vi "Acquire Sound.vi"() -> (0 "DAQ Error":errorcluster)   [LabVIEW 2021]
uses:
  Sub_vis/Upload Data.ctl
  Globals/Meas_global.vi
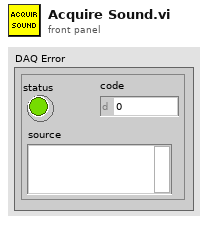
[diagram p1: front panel]
types:
  T1 = typedef "Setup.ctl" = enum16{"Run Program", "Show Setup", "Save Current Setup", "Setup Front Panel"}
  T2 = typedef "Upload Data.ctl" = enum16{"Voltage Array", "Time Trace Cluster"}
  T3 = typedef "Analysis_info_cluster.ctl" = cluster{"Colour":u32, "Inst type":T4, "Inst name":string, "Symbol":string, "Code name":string, "Extra Info":string, "Inst Array":T5, "Extra Titles":string[], "Extra Values":string[], "U":dbl, "u^2":dbl, "u^3":dbl, "u^4":dbl, "Skew_u":dbl, "Kurt_u":dbl, "Sd Error in Mean":dbl, "% u'/U":dbl, "X":dbl, "Y":dbl, "Z":dbl, "Timescale integral Estimate":dbl, "Sd Error in Variance":dbl, "Calib File":path, "Calib Constants":dbl[], "Output Position":bool, "Stats":enum16{"None", "Basic", "Full"}, "Av Sampling Rate":dbl, "Av No of Samples":dbl, "Total Meas Time (s)":dbl, "ADAM Ch Name":string, "Max value":dbl, "Min value":dbl, "Req Sample Rate Hz":dbl, "Sync Delay Time (s)":dbl, "Ch No":i16, "Device":string, "Use Latest Calib":bool, "Port":string, "Metadata Ch Names":string[], "Metadata Ch Values":string[], "Label":string}
  T4 = typedef "Inst_type.ctl" = enum16{"Raw voltage", "Raw with zero offsetting", "Propeller anemometer", "Pressure Transducer", "Pitot-static tube", "Hot wire", "Cross wire 1", "Cross wire 2", "Generic Linear", "Generic Polynomial", "Generic BackPoly", "Fast FID", "Thermocouple", "Cold wire", "Pulsed Wire", "LDA Vel", "LDA Tran time", "LDA Arr time", "Microphone"}
  T5 = typedef "Instrument_Array.ctl" = enum16{"PWA", "LDA", "Analogue"}
  T6 = typedef "Device ID port info.ctl" = cluster{"Ch No":i16[], "Req Sampling Rate":dbl[], "Port":string, "Index":i32[]}
  T7 = typedef "Rendezvous RefNum" = refnum<k1>
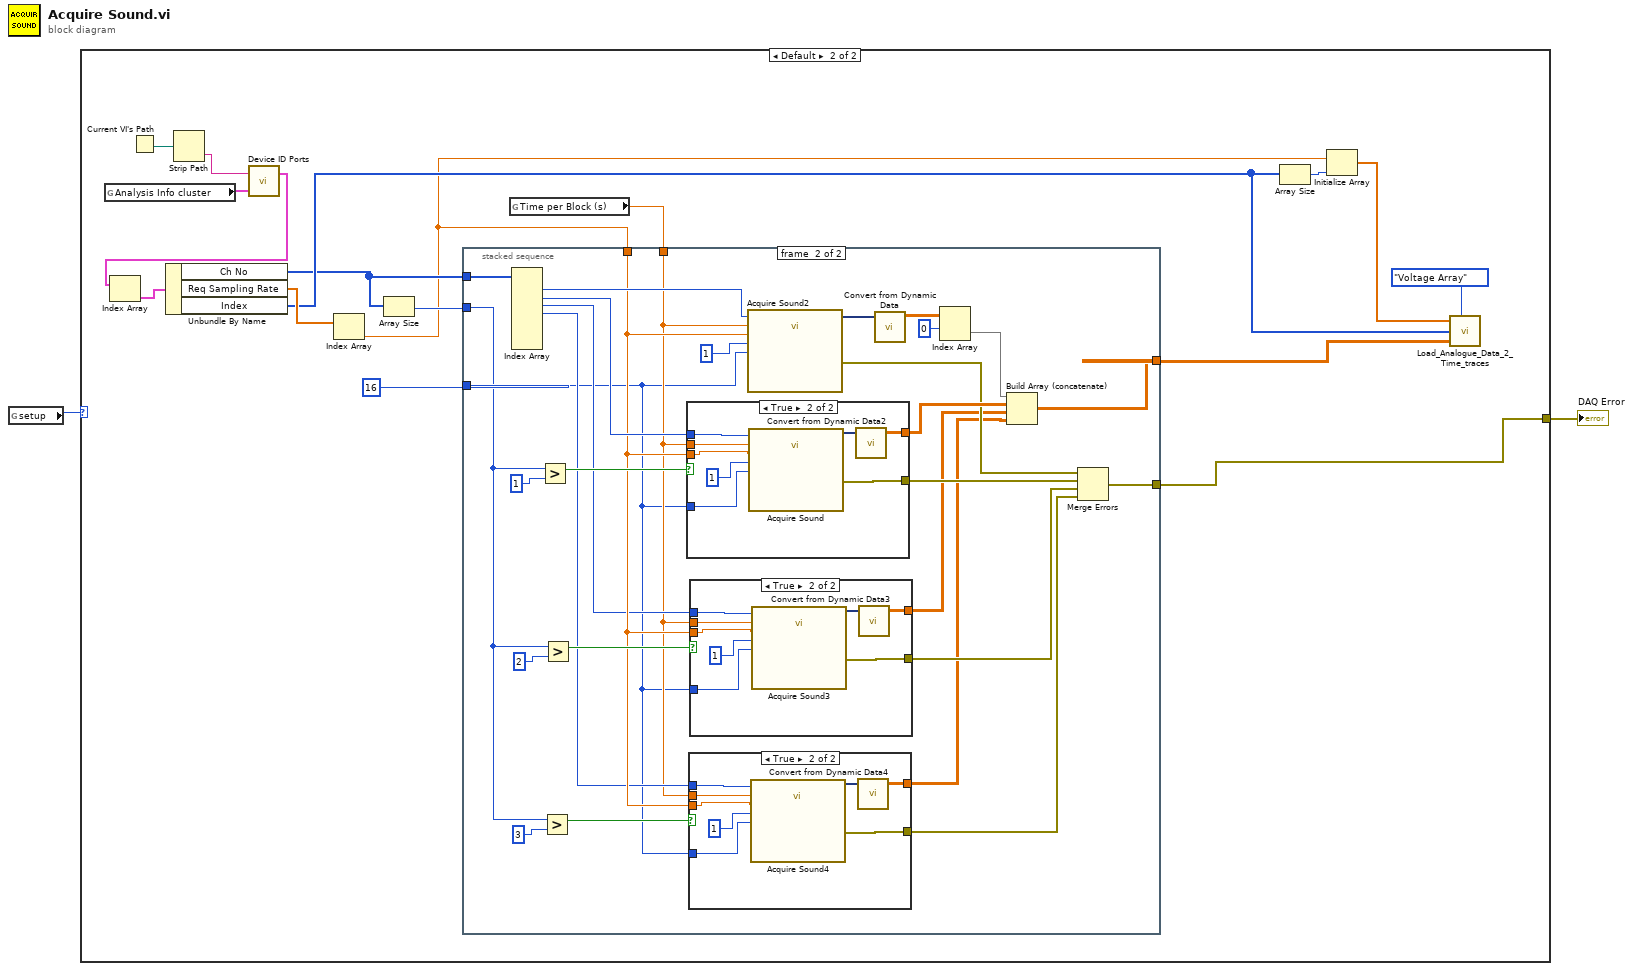
[diagram p0: block diagram]
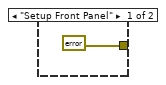
[diagram p2: hidden frame]
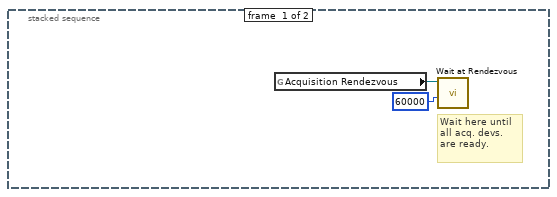
[diagram p3: hidden frame]
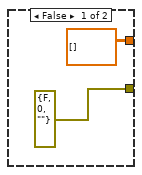
[diagram p4: hidden frame]
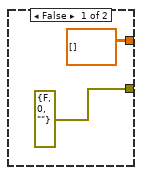
[diagram p5: hidden frame]
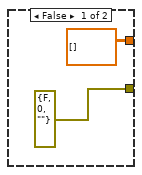
[diagram p6: hidden frame]
diagram:
  n1 = global read "Meas_global.vi" "setup"() -> (w2:T1)
  n2 = case shown="Default" w2 {
    tunnel: [errorcluster {"status"=FALSE, "code"=0, "source"=""} ("DAQ Error") w4] -> w1
    frame "Setup Front Panel" {
    }
    frame Default {
      n3 = global read "Meas_global.vi" "Analysis Info cluster"() -> (w18:T3[])
      n4 = Current VI's Path() -> (path=w20:path)
      n5 = Strip Path(path=w20) -> (name=w19:string)  [unwired: 1 out]
      n6 = call "Device ID Ports.vi"("Analysis Info cluster"=w18, "Device ID"=w19) -> ("Device port info"=w17:T6[])  [unwired: 1 out]
      n7 = Index Array(array=w17) -> (element=w16:T6)  [unwired: 1 in]
      n8 = Unbundle By Name(w16) -> ("Ch No"=w6:i16[], "Req Sampling Rate"=w14:dbl[], "Index"=w10:i32[])
      n9 = Index Array(array=w14) -> (element=w5:dbl)  [unwired: 1 in]
      n10 = Array Size(array=w6) -> (size(s)=w8:i32)
      n11 = global read "Meas_global.vi" "Time per Block (s)"() -> (w7:dbl)
      n12 = stacked-sequence {
        tunnel: 16 ("Resolution (bits)") -> [_ w23]
        tunnel: [_ w26] -> w12
        tunnel: w8 -> [_ w34]
        tunnel: w7 -> [_ w30]
        tunnel: w6 -> [_ w48]
        tunnel: w5 -> [_ w33]
        tunnel: [_ w27] -> w4
        frame #0 {
          # "Wait here until all acq. devs. are ready."
          n13 = global read "Meas_global.vi" "Acquisition Rendezvous"() -> (w22:T7)
          n14 = call <vilib>:"Wait at Rendezvous.vi"("ms timeout (-1)"=60000, "rendezvous"=w22) -> ()  [unwired: 3 in, 3 out]
        }
        frame #1 {
          n15 = Index Array(array=w48) -> (element #1=w47:i16, element #2=w46:i16, element #3=w32:i16, element #4=w31:i16)  [unwired: 8 in, 4 out]
          n16 = Greater?(x=w34, y=1) -> (0:w49:bool)
          n17 = Greater?(x=w34, y=3) -> (0:w35:bool)
          n18 = Greater?(x=w34, y=2) -> (0:w38:bool)
          n19 = case shown="True" w49 {
            tunnel: w46 -> [_ w80]
            tunnel: w30 -> [_ w79]
            tunnel: w33 -> [_ w78]
            tunnel: [dbl[][] [] ("Array") w76] -> w41
            tunnel: [errorcluster {"status"=FALSE, "code"=0, "source"=""} ("error out") w75] -> w39
            tunnel: w23 -> [_ w74]
            frame False {
            }
            frame True {
              n20 = call "Acquire Sound"("Device"=w80, "Duration (s)"=w79, "Sample rate (Hz)"=w78, "#Channels"=1, "Resolution (bits)"=w74) -> ("Data"=w77:dynamicdata, "error out"=w75:errorcluster)  [unwired: 13 in]
              n21 = call "Convert from Dynamic Data2"("Dynamic Data Type"=w77) -> ("Array"=w76:dbl[][])  [unwired: 3 in]
            }
          }
          n22 = case shown="True" w35 {
            tunnel: w31 -> [_ w60]
            tunnel: w30 -> [_ w59]
            tunnel: w33 -> [_ w58]
            tunnel: [dbl[][] [] ("Array") w56] -> w24
            tunnel: [errorcluster {"status"=FALSE, "code"=0, "source"=""} ("error out") w55] -> w28
            tunnel: w23 -> [_ w54]
            frame False {
            }
            frame True {
              n23 = call "Acquire Sound4"("Device"=w60, "Duration (s)"=w59, "Sample rate (Hz)"=w58, "#Channels"=1, "Resolution (bits)"=w54) -> ("Data"=w57:dynamicdata, "error out"=w55:errorcluster)  [unwired: 13 in]
              n24 = call "Convert from Dynamic Data4"("Dynamic Data Type"=w57) -> ("Array"=w56:dbl[][])  [unwired: 3 in]
            }
          }
          n25 = case shown="True" w38 {
            tunnel: w32 -> [_ w70]
            tunnel: w30 -> [_ w69]
            tunnel: w33 -> [_ w68]
            tunnel: [dbl[][] [] ("Array") w66] -> w25
            tunnel: [errorcluster {"status"=FALSE, "code"=0, "source"=""} ("error out") w65] -> w29
            tunnel: w23 -> [_ w64]
            frame False {
            }
            frame True {
              n26 = call "Acquire Sound3"("Device"=w70, "Duration (s)"=w69, "Sample rate (Hz)"=w68, "#Channels"=1, "Resolution (bits)"=w64) -> ("Data"=w67:dynamicdata, "error out"=w65:errorcluster)  [unwired: 13 in]
              n27 = call "Convert from Dynamic Data3"("Dynamic Data Type"=w67) -> ("Array"=w66:dbl[][])  [unwired: 3 in]
            }
          }
          n28 = call "Acquire Sound2"("Device"=w47, "Duration (s)"=w30, "Sample rate (Hz)"=w33, "#Channels"=1, "Resolution (bits)"=w23) -> ("Data"=w45:dynamicdata, "error out"=w40:errorcluster)  [unwired: 13 in]
          n29 = call "Convert from Dynamic Data"("Dynamic Data Type"=w45) -> ("Array"=w43:dbl[][])  [unwired: 3 in]
          n30 = Index Array(array=w43, index (row)=0) -> (element=w42:dbl[])  [unwired: 1 in]
          n31 = Build Array (concatenate)(w42, w41, w25, w24) -> (w26:dbl[][])
          n32 = Merge Errors(w40, w39, w29, w28) -> (w27:errorcluster)
        }
      }
      n33 = Array Size(array=w10) -> (size(s)=w11:i32)
      n34 = Initialize Array(w5, w11) -> (w9:dbl[])
      n35 = call "Load_Analogue_Data_2_Time_traces.vi"("Sampling Rate (Hz)"=w9, "Mode"=Upload_Data."Voltage Array", "Index"=w10, "Voltage Array"=w12) -> ()  [unwired: 3 in]
    }
  }
  "DAQ Error" <- w1
